vi "Schedule List.vi"() -> (3 "schedules":string[](array[string]))   [LabVIEW 2019, in "Pet Feeder.lvlib"]
uses:
  Pet Feeder.lvlib
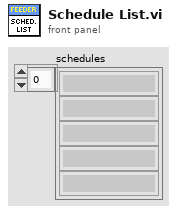
[diagram p1: front panel]
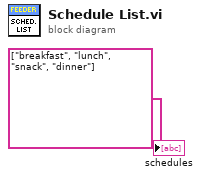
[diagram p0: block diagram]
diagram:
  "schedules" <- string[] ["breakfast", "lunch", "snack", "dinner"]
